vi "Pre Launch Init.vi"(11 "Nested in":refnum<class "UI Actor.lvclass">) -> (0 "error out":errorcluster, 3 "Nested out":refnum<class "UI Actor.lvclass">)   [LabVIEW 2020, in "UI Actor.lvlib" / "UI Actor.lvclass"]
doc: "(<B>Filename</B>: Actor Framework.lvlib:Actor.lvclass:Pre Launch Init.vi)\n\nDefines behavior that occurs after the Launch Nested Actor method is invoked but before the actor's Actor Core method begins running.\n\nBy default, this method does nothing. A descendant class may override it to define behavior."
uses:
  UI Actor.lvclass
  C:/Program Files (x86)/National Instruments/LabVIEW 2020/vi.lib/ActorFramework/Actor/Actor.lvclass
  UI Actor.lvclass/UI Actor.ctl
  <vilib>/ActorFramework/Actor/Actor.lvclass/Actor.ctl
  <vilib>/ActorFramework/Message Enqueuer/Message Enqueuer.lvclass/Message Enqueuer.ctl
  <vilib>/ActorFramework/Message Enqueuer/Init from Existing Queue.vi
  <vilib>/ActorFramework/Message Enqueuer/Enqueue.vi
  UI Actor Messages/Init Msg/Init Msg.lvclass
  C:/Program Files (x86)/National Instruments/LabVIEW 2020/vi.lib/ActorFramework/Message/Message.lvclass
  <vilib>/ActorFramework/Message Priority Queue/Priority Enqueue.vi
  <vilib>/ActorFramework/Message Enqueuer/Message Enqueuer.lvclass
  <vilib>/ActorFramework/Actor/Actor.lvclass
  C:/Users/Asus/Dropbox/trabajos_apuntes/7 semestre/labview/Actor Framework 2 Parcial/UI Actor/UI Actor.lvclass
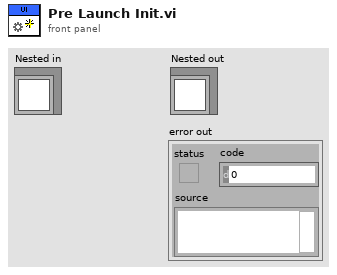
[diagram p1: front panel]
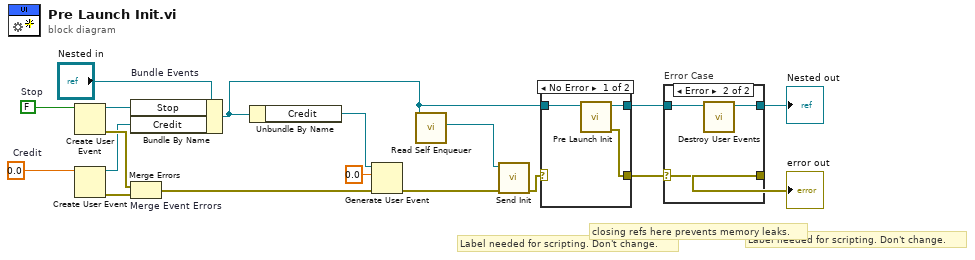
[diagram p0: block diagram]
diagram:
  w8 = 0.0  # Credit
  w17 = FALSE  # Stop
  # "Label needed for scripting. Don't change."
  # "Label needed for scripting. Don't change."
  # "closing refs here prevents memory leaks."
  n1 = Create User Event(user event datatype=w17) -> (user event=w14:refnum<user-event>, error out=w16:errorcluster)  [unwired: 1 in]
  n2 = Create User Event(user event datatype=w8) -> (user event=w7:refnum<user-event>, error out=w6:errorcluster)  [unwired: 1 in]
  n3 = Bundle By Name "Bundle Events"(cluster="Nested in", "Stop"=w14, "Credit"=w7) -> (w5:refnum<class "UI Actor.lvclass">)
  n4 = Merge Errors "Merge Event Errors"(w16, w6) -> (w4:errorcluster)
  n5 = Unbundle By Name(w5) -> ("Credit"=w2:refnum<user-event>)
  n6 = Generate User Event(user event=w2, event data cluster=0.0 ("event data"), error in=w4) -> (error out=w3:errorcluster)  [unwired: 1 in, 1 out]
  n7 = call <vilib>:"Read Self Enqueuer.vi"("Actor"=w5) -> ("Self Enqueuer"=w10:refnum<class "Message Enqueuer.lvclass">)  [unwired: 10 in]
  n8 = call "Send Init.vi"("error in (no error)"=w3, "Message Enqueuer"=w10) -> ("error out"=w9:errorcluster)  [unwired: 8 in, 1 out]
  n9 = case shown="No Error" w9 {
    selector: w9 -> [_ w23]
    tunnel: [w21 w22] -> w12
    tunnel: w5 -> [w20 w22]
    tunnel: [w19 w23] -> w11
    frame No Error {
      n10 = call-parent "Pre Launch Init.vi"("Actor in"=w20) -> ("error out"=w19:errorcluster, "Actor out"=w21:refnum<class "UI Actor.lvclass">)  [unwired: 9 in]
    }
    frame Error {
    }
  }
  n11 = case "Error Case" shown="Error" w11 {
    selector: w11 -> [w24 w28]
    tunnel: w12 -> [w25 w27]
    tunnel: [w25 w26] -> w15
    tunnel: [w24 w28] -> w13
    frame No Error {
    }
    frame Error {
      n12 = call "Destroy User Events.vi"("UI Template in"=w27) -> ("UI Template out"=w26:refnum<class "UI Actor.lvclass">)  [unwired: 10 in]
    }
  }
  "error out" <- w13
  "Nested out" <- w15
